vi "test bishop.vi"() -> ()   [LabVIEW 2016]
uses:
  Chesslib/Moves/Move/Move.lvclass
  Chesslib/typedef/Square.ctl
  Chesslib/typedef/File.ctl
  Chesslib/typedef/Rank.ctl
  Chesslib/typedef/Piece type.ctl
  Chesslib/typedef/Color.ctl
  Chesslib/Position/Position.lvclass/Position.ctl
  Chesslib/Pieces/Piece/Piece.lvclass
  Chesslib/Position/Position.lvclass
  Chesslib/Board/Board.lvclass
  Chesslib/Chesslib.lvlib
panel:
  out "size(s)":i32
  out "Moves":refnum<class "Move.lvclass">[](array[class])
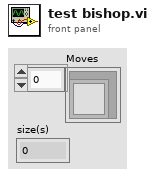
[diagram p1: front panel]
types:
  T1 = typedef "Chesslib.lvlib/Square.ctl" = cluster{"File":T2, "Rank":T3}
  T2 = typedef "Chesslib.lvlib/File.ctl" = enum8{"a", "b", "c", "d", "e", "f", "g", "h"}
  T3 = typedef "Chesslib.lvlib/Rank.ctl" = enum8{"1", "2", "3", "4", "5", "6", "7", "8"}
  T4 = typedef "Chesslib.lvlib/Color.ctl" = enum16{"White", "Black"}
  T5 = typedef "Chesslib.lvlib/Piece type.ctl" = enum16{"Pawn", "Bishop", "Knight", "Rook", "Queen", "King"}
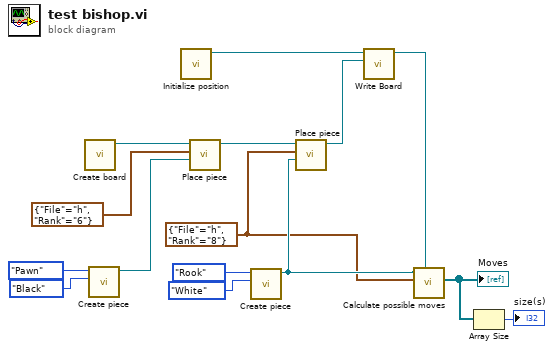
[diagram p0: block diagram]
diagram:
  w9 = T1 {"File"=enum."h", "Rank"=enum."8"} ("Square")
  n1 = call "Create board.vi"() -> ("Empty board"=w14:refnum<class "Board.lvclass">)  [unwired: 11 in]
  n2 = call "Create piece.vi"("Piece color"=Color."Black", "Piece type"=Piece_type."Pawn") -> ("Piece out"=w2:refnum<class "Piece.lvclass">)  [unwired: 9 in]
  n3 = call "Initialize position.vi"() -> ("Position out"=w15:refnum<class "Position.lvclass">)  [unwired: 10 in, 1 out]
  n4 = call "Place piece.vi"("Piece"=w2, "Square"=T1 {"File"=enum."h", "Rank"=enum."6"}, "Board in"=w14) -> ("Board out"=w5:refnum<class "Board.lvclass">)  [unwired: 6 in, 2 out]
  n5 = call "Create piece.vi"("Piece color"=Color."White", "Piece type"=Piece_type."Rook") -> ("Piece out"=w10:refnum<class "Piece.lvclass">)  [unwired: 9 in]
  n6 = call "Place piece.vi"("Piece"=w10, "Square"=w9, "Board in"=w5) -> ("Board out"=w11:refnum<class "Board.lvclass">)  [unwired: 6 in, 2 out]
  n7 = call "Write Board.vi"("Board"=w11, "Position in"=w15) -> ("Position out"=w8:refnum<class "Position.lvclass">)  [unwired: 9 in]
  n8 = call-dynamic "Calculate possible moves.vi"("Position"=w8, "Source"=w9, "Piece in"=w10) -> ("Moves"=w7:refnum<class "Move.lvclass">[])  [unwired: 6 in, 2 out]
  "Moves" <- w7
  n9 = Array Size(array=w7) -> (size(s)=→"size(s)":i32)
